vi "Set RPC getCANDatafromrgrpcServer_clientRequester_getIDFormServer __Output.vi"(7 "Streeming? (F)":bool, 8 "error in (no error)":errorcluster, 10 "Message Data":T1, 11 "gRPCid in":T2) -> (0 "error out":errorcluster)   [LabVIEW 2020, in "server1.lvlib" / "server1.lvclass"]
uses:
  server1.lvclass
  gRPC lvSupport/Server API/typeDefs/grpcId.ctl
  server1.lvclass/server1.ctl
  gRPC lvSupport/gprc-lvsupport.lvlib
  RPC Messages/getCANDatafromrgrpcServer_getFrameResponse/getCANDatafromrgrpcServer_getFrameResponse_Data.ctl
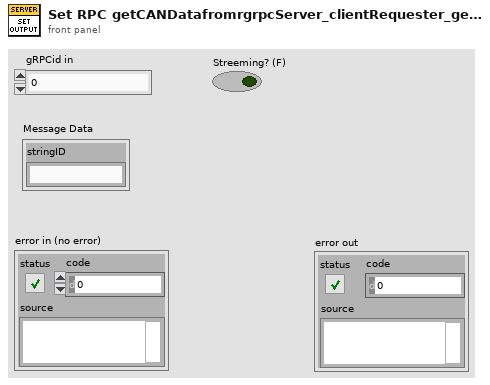
[diagram p1: front panel]
types:
  T1 = typedef "server1.lvlib/server1.lvclass/getCANDatafromrgrpcServer_getFrameResponse_Data.ctl" = cluster{"stringID":string}
  T2 = typedef "server1.lvlib/gprc-lvsupport.lvlib/grpcId.ctl" = u64
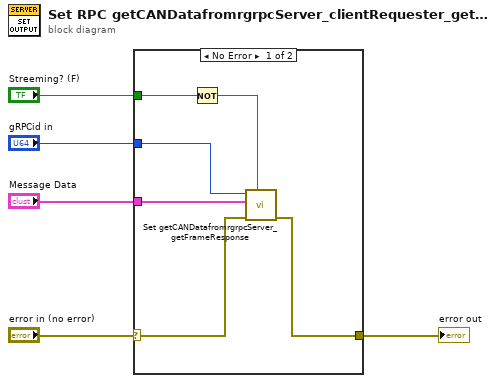
[diagram p0: block diagram]
diagram:
  n1 = case shown="No Error" "error in (no error)" {
    selector: "error in (no error)" -> [w11 w12]
    tunnel: [w9 w12] -> w4
    tunnel: "gRPCid in" -> [w10 _]
    tunnel: "Message Data" -> [w8 _]
    tunnel: "Streeming? (F)" -> [w7 _]
    frame No Error {
      n2 = Not(x=w7) -> (.not. x?=w6:bool)
      n3 = call "Set getCANDatafromrgrpcServer_getFrameResponse.vi"("Complete Call (T)"=w6, "error in (no error)"=w11, "Message Data"=w8, "gRPCid"=w10) -> ("error out"=w9:errorcluster)  [unwired: 7 in]
    }
    frame Error {
    }
  }
  "error out" <- w4
